vi "programa 13.vi"() -> ()   [LabVIEW 2011]
panel:
  in  "stop":bool
  out "Velocidad":dbl(knob) scale=0.0..180.0
  in  "Reducir":bool
  in  "Aumentar":bool
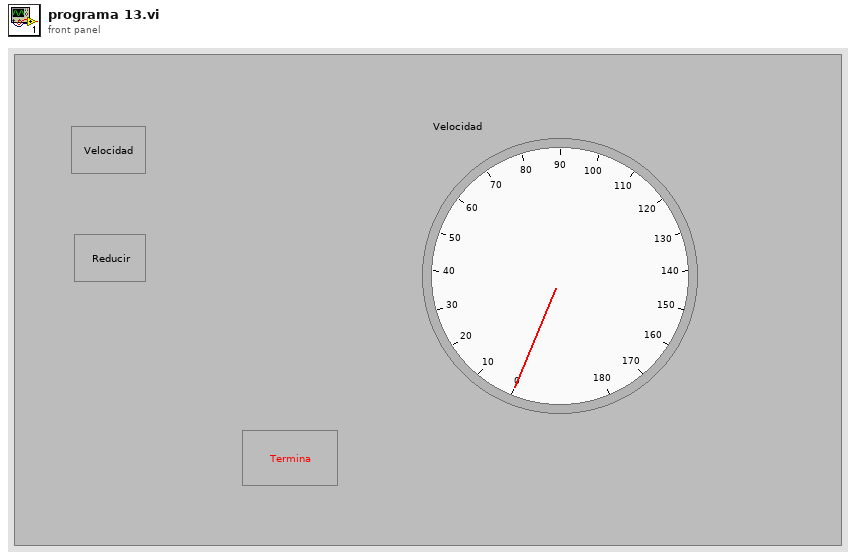
[diagram p1: front panel]
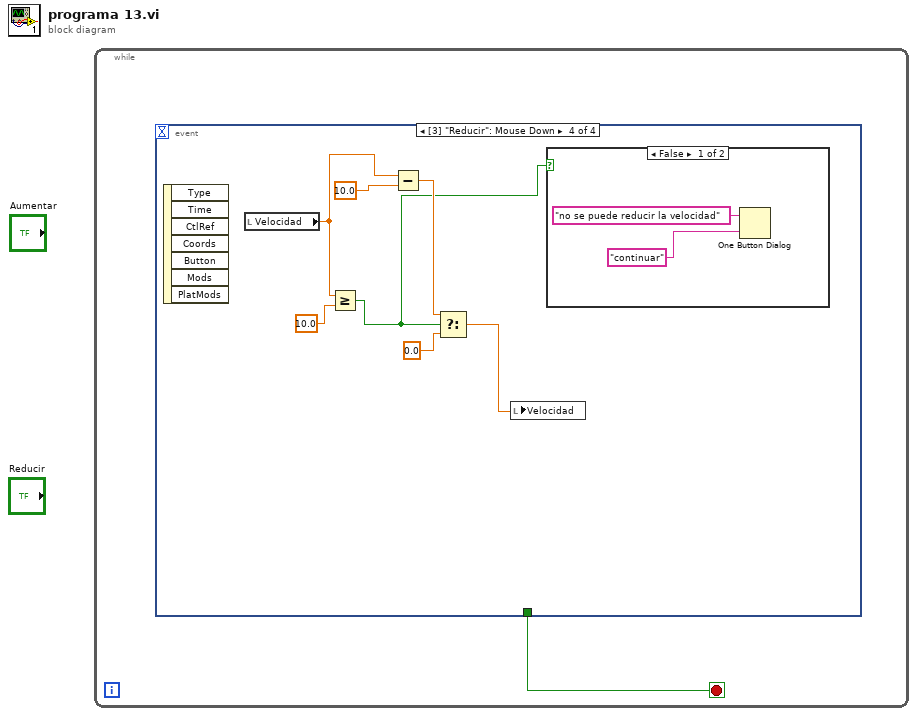
[diagram p0: block diagram]
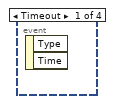
[diagram p2: hidden frame]
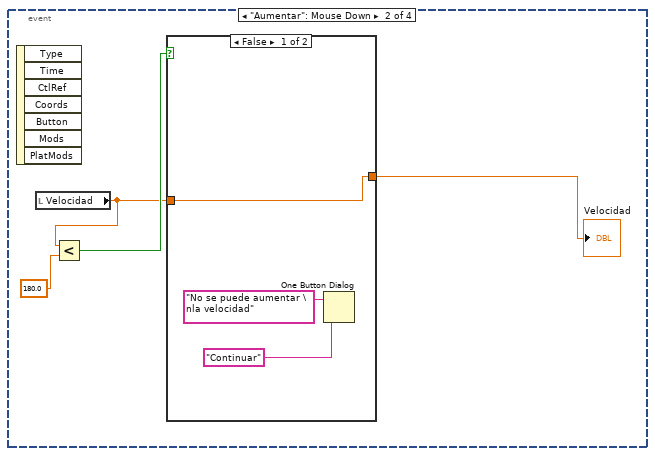
[diagram p3: hidden frame]
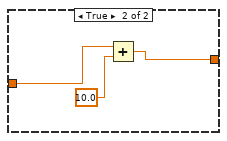
[diagram p4: hidden frame]
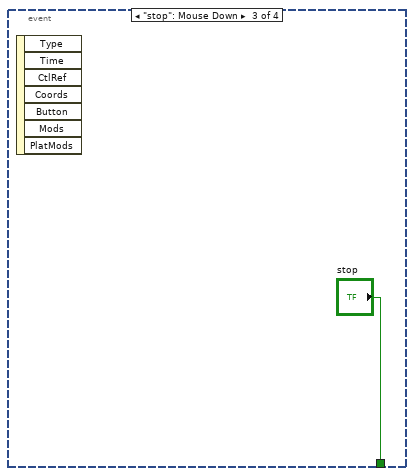
[diagram p5: hidden frame]
diagram:
  n1 = while {
    stop <- w1 stop-if-true
    n2 = event shown="[3] \"Reducir\": Mouse Down" {
      selector: _ -> [_ _ _ _]
      dyn-events: _ -> [_ _ _ _]
      timeout: _ -> [_ _ _ _]
      tunnel: [_ _ "stop" _] -> w1
      event Timeout {
        n3 = event-data() -> ()  [unwired: 1 in, 2 out]
      }
      event "Aumentar": Mouse Down {
        n4 = event-data() -> ()  [unwired: 1 in, 7 out]
        n5 = local read "Velocidad"() -> (w3:dbl)
        n6 = Less?(x=w3, y=180.0) -> (x < y?=w4:bool)
        n7 = case shown="False" w4 {
          tunnel: w3 -> [w8 w11]
          tunnel: [w8 w9] -> w2
          frame False {
            n8 = One Button Dialog(message="No se puede aumentar \nla velocidad", button name ("OK")="Continuar") -> ()  [unwired: 1 out]
          }
          frame True {
            n9 = Add(x=w11, y=10.0) -> (x+y=w9:dbl)
          }
        }
        "Velocidad" <- w2
      }
      event "stop": Mouse Down {
        n10 = event-data() -> ()  [unwired: 1 in, 7 out]
      }
      event "Reducir": Mouse Down {
        n11 = event-data() -> ()  [unwired: 1 in, 7 out]
        n12 = local read "Velocidad"() -> (w15:dbl)
        n13 = Greater Or Equal?(x=w15, y=10.0) -> (x >= y?=w13:bool)
        n14 = Subtract(x=w15, y=10.0) -> (x-y=w14:dbl)
        n15 = Select(t=w14, s=w13, f=0.0 ("y")) -> (s? t:f=w17:dbl)
        n16 = local write "Velocidad"(w17) -> ()
        n17 = case shown="False" w13 {
          frame False {
            n18 = One Button Dialog(message="no se puede reducir la velocidad", button name ("OK")="continuar") -> ()  [unwired: 1 out]
          }
          frame True {
          }
        }
      }
    }
  }
